vi "Create.vi"(8 "error in (no error)":errorcluster, 11 "group count (1)":u64=1) -> (0 "error out":errorcluster, 3 "Transfer Group Status":refnum<class "Transfer Group Status.lvclass">)   [LabVIEW 2017, in "DSF Core.lvlib" / "Transfer Group Status.lvclass"]
uses:
  Transfer Group Status.lvclass
  C:/Program Files (x86)/National Instruments/LabVIEW 2017/vi.lib/NI/Memory Manager/Classes/Pointer/Pointer.lvclass
  Typedefs/DSF Transfer Group Status.ctl
  <vilib>/NI/Memory Manager/Classes/Pointer/Pointer.lvclass/Pointer.ctl
  <vilib>/NI/Memory Manager/Classes/Pointer/Set Address.vi
  <vilib>/NI/Memory Manager/Classes/Pointer/Set Size.vi
  <vilib>/NI/Memory Manager/Classes/Pointer/Set Internal.vi
  <vilib>/NI/Memory Manager/Classes/Pointer/Check Size (0D).vi
  <vilib>/NI/Memory Manager/Classes/Pointer/Get Address.vi
  <vilib>/NI/Memory Manager/Classes/Pointer/Errors.vi
  <vilib>/NI/Memory Manager/Classes/Pointer/Out of Bounds.vi
  <vilib>/NI/Memory Manager/Classes/Pointer/Get Size.vi
  <vilib>/NI/Memory Manager/VIs/Source.Write.String.vi
  <vilib>/NI/Memory Manager/Classes/Pointer/Write Pointer Size.vi
  <vilib>/NI/Memory Manager/Classes/Pointer/Create Error.vi
  <vilib>/NI/Memory Manager/VIs/Source.Write.Scalar.Base10.vi
  <vilib>/NI/Memory Manager/VIs/Source.Write.Scalar.Base10 (U64).vi
  <vilib>/NI/Memory Manager/VIs/New Error Cluster Constant.vi
  <vilib>/NI/Memory Manager/VIs/New Error Cluster Constant (512B).vi
  <vilib>/NI/Memory Manager/VIs/Error Cluster.Set Status.vi
  <vilib>/NI/Memory Manager/VIs/Error Cluster.Set Code.vi
  <vilib>/NI/Memory Manager/VIs/Error Cluster.Set VI Source.vi
  <vilib>/NI/Memory Manager/Constants/Constants.vi
  <vilib>/NI/Memory Manager/Constants/Library Name.vi
  <vilib>/NI/Memory Manager/Classes/Pointer/Pointer Error Info.vi
  <vilib>/NI/Memory Manager/Constants/Pointer Class Name.vi
  DSF Core.lvlib
  <vilib>/NI/Memory Manager/Classes/Pointer/Pointer.lvclass
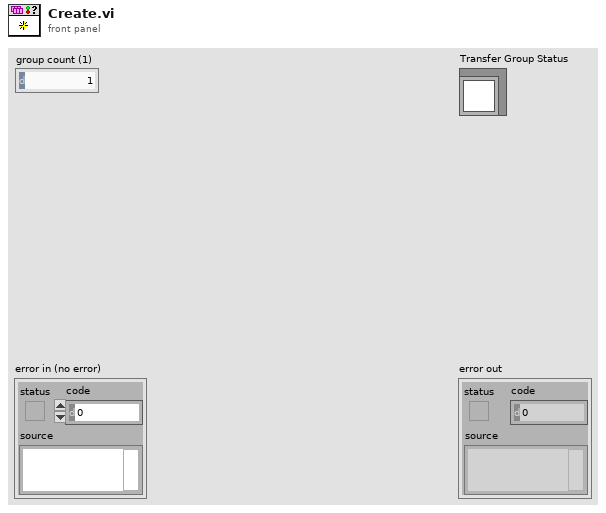
[diagram p1: front panel]
types:
  T1 = typedef "DSF Core.lvlib/DSF Transfer Group Status.ctl" = cluster{"late count":u64, "iteration":u64}
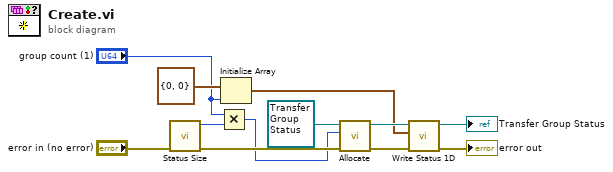
[diagram p0: block diagram]
diagram:
  n1 = call "Status Size.vi"("error in (no error)"="error in (no error)") -> ("error out"=w5:errorcluster, "size"=w8:u64)  [unwired: 9 in]
  n2 = Multiply(x="group count (1)", y=w8) -> (x*y=w1:u64)
  n3 = Initialize Array(T1 {"late count"=0, "iteration"=0} ("Transfer Group status"), "group count (1)") -> (w2:T1[])
  n4 = call <vilib>:"Allocate.vi"("error in (no error)"=w5, "size"=w1, "Pointer in"=refnum<class "Transfer Group Status.lvclass"> refnum ("Transfer Group Status in")) -> ("error out"=w4:errorcluster, "Pointer out"=w3:refnum<class "Transfer Group Status.lvclass">)  [unwired: 7 in]
  n5 = call "Write Status 1D.vi"("error in (no error)"=w4, "status"=w2, "Transfer Group Status in"=w3) -> ("error out"=→"error out":errorcluster, "Transfer Group Status out"=→"Transfer Group Status":refnum<class "Transfer Group Status.lvclass">)  [unwired: 7 in]
